vi "feedbackarrow.vi"() -> ()   [LabVIEW 2017]
panel:
  out "Nodo fuera":dbl
  out "Nodo dentro":dbl
  in  "Numero a\nsumar":dbl=14.0
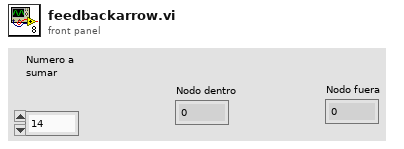
[diagram p1: front panel]
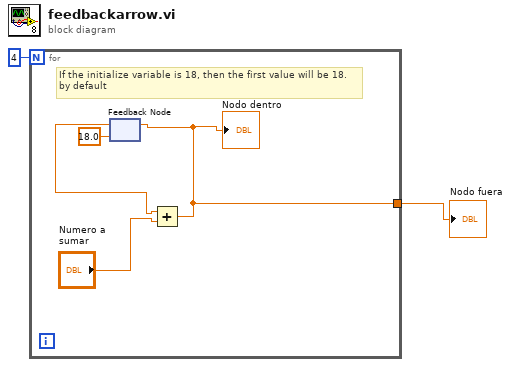
[diagram p0: block diagram]
diagram:
  n1 = for {
    N: 4 -> [_]
    tunnel: [w4] -> w2
    # "If the initialize variable is 18, then the first value will be 18.\nby default"
    n2 = feedback #1(18.0) -> (w5:dbl)
    n3 = Add(x=w5, y="Numero a\nsumar") -> (x+y=w4:dbl)
    "Nodo dentro" <- w4
    n4 = feedback-in #1(w4) -> ()
  }
  "Nodo fuera" <- w2
